vi "Location Analysis.vi"(3 "error in (no error)":errorcluster, 4 "Microphone Locations":cluster{"r":dbl, "theta":dbl, "z":dbl}[](array[cluster]), 5 "Signals":waveform(dbl)[](array[waveform])) -> (0 "error out":errorcluster)   [LabVIEW 2013, in "Breakdown Acoustics Controls.lvlib"]
uses:
  Breakdown Acoustics Controls.lvlib
panel:
  out "Distance from Known Coordinates":dbl[](array[numeric])
  out "Known Coordinates (cm, cm, cm)":cluster{"x":dbl, "y":dbl, "z":dbl}[](array[cluster])
  in  "Known Coordinates (cm, rad, cm)":cluster{"r":sgl, "theta":sgl, "z":sgl}[](array[cluster])
  out "Cavity Downstream View":refnum<vi>(3d-picture)
  out "Coordinates (cm, cm, cm)":cluster{"x":dbl, "y":dbl, "z":dbl}[](array[cluster])
  in  "Correlation Region (ms)":cluster{dbl, dbl}(slide)={0.9, 0.6} scale=0.0..2.0
  out "Coordinates (cm, rad, cm)":cluster{"r":sgl, "theta":sgl, "z":sgl}[](array[cluster])
  out "Cavity Side (codirectional with x) View":refnum<vi>(3d-picture)
  out "Cavity Upstream View":refnum<vi>(3d-picture)
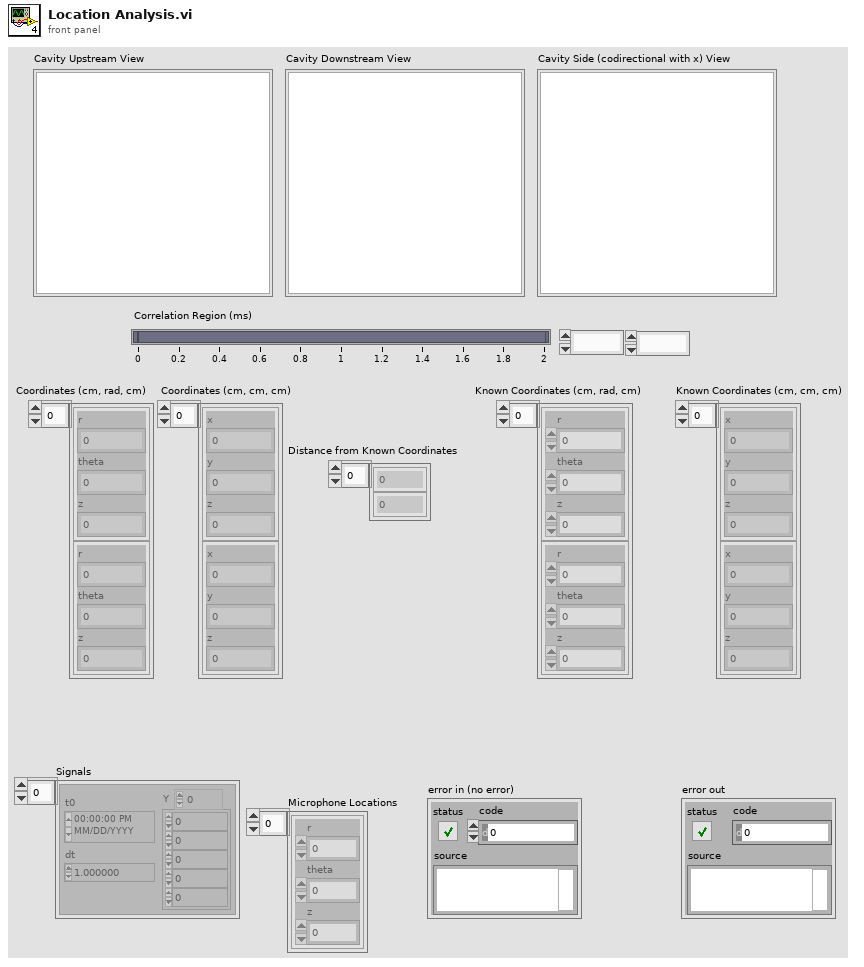
[diagram p1: front panel]
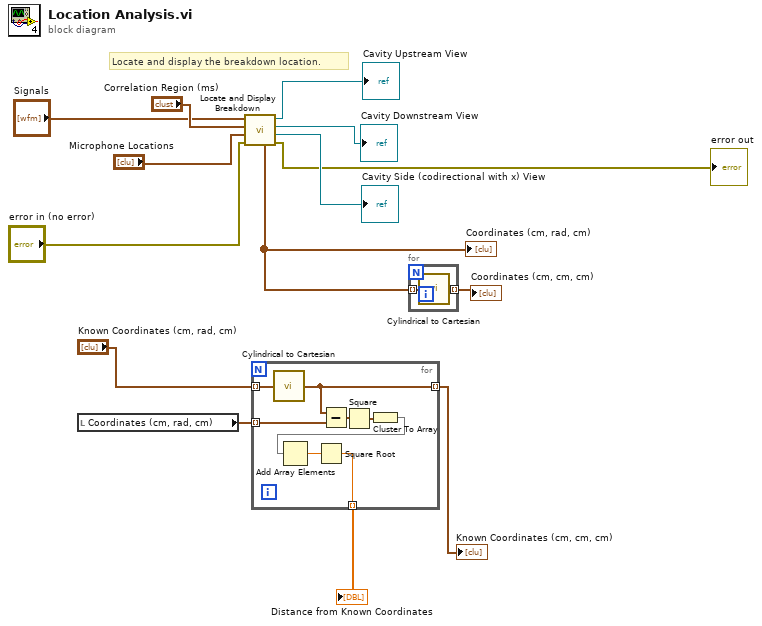
[diagram p0: block diagram]
diagram:
  # "Locate and display the breakdown location."
  n1 = local read "Coordinates (cm, rad, cm)"() -> (w2:cluster{"r":sgl, "theta":sgl, "z":sgl}[])
  n2 = call "Locate and Display Breakdown.vi"("error in (no error)"="error in (no error)", "Microphone Locations"="Microphone Locations", "Correlation Region (ms)"="Correlation Region (ms)", "Signals"="Signals") -> ("error out"=→"error out":errorcluster, "Side View Scene"=→"Cavity Side (codirectional with x) View":refnum<vi>, "Downstream View Scene"=→"Cavity Downstream View":refnum<vi>, "Upstream View Scene"=→"Cavity Upstream View":refnum<vi>, "Coordinates (cm, rad, cm)"=w13:cluster{"r":sgl, "theta":sgl, "z":sgl}[])  [unwired: 3 in]
  "Coordinates (cm, rad, cm)" <- w13
  n3 = for {
    tunnel: "Known Coordinates (cm, rad, cm)" -> [w22] mode=indexing
    tunnel: [w21] -> w3 mode=indexing
    tunnel: w2 -> [w19] mode=indexing
    tunnel: [w15] -> w1 mode=indexing
    n4 = call "Cylindrical to Cartesian.vi"("Cylindrical\nCoordinates"=w22) -> ("Cartesian\nCoordinates"=w21:cluster{"x":dbl, "y":dbl, "z":dbl})  [unwired: 4 in]
    n5 = Subtract(x=w21, y=w19) -> (x-y=w20:cluster{dbl, dbl, "z":dbl})
    n6 = Square(x=w20) -> (x^2=w18:cluster{dbl, dbl, "z":dbl})
    n7 = Cluster To Array(cluster=w18) -> (array=w17:dbl[])
    n8 = Add Array Elements(numeric array=w17) -> (sum=w16:dbl)
    n9 = Square Root(x=w16) -> (sqrt(x)=w15:dbl)
  }
  "Known Coordinates (cm, cm, cm)" <- w3
  "Distance from Known Coordinates" <- w1
  n10 = for {
    tunnel: w13 -> [w24] mode=indexing
    tunnel: [w23] -> w14 mode=indexing
    n11 = call "Cylindrical to Cartesian.vi"("Cylindrical\nCoordinates"=w24) -> ("Cartesian\nCoordinates"=w23:cluster{"x":dbl, "y":dbl, "z":dbl})  [unwired: 4 in]
  }
  "Coordinates (cm, cm, cm)" <- w14
